vi "GetIndexInRange.vi"(8 "location":u32, 9 "buffer size":u32, 10 "last block":u32, 11 "write pointer":i32) -> (1 "index":i32, 2 "in range":bool)   [LabVIEW 2017, in "DVRBuffer.lvlib"]
uses:
  <vilib>/addons/InsightCM/Devices/Shared/Common/DVRBuffer/DVRBuffer.lvlib
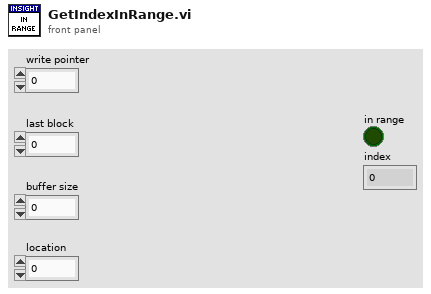
[diagram p1: front panel]
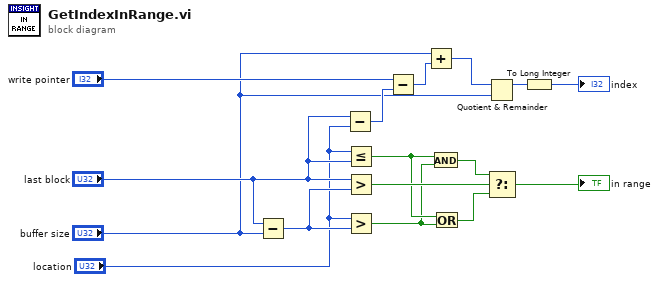
[diagram p0: block diagram]
diagram:
  n1 = Subtract(x="last block", y="buffer size") -> (x-y=w16:u32)
  n2 = Subtract(x="last block", y="location") -> (x-y=w14:u32)
  n3 = Less Or Equal?(x="location", y="last block") -> (x <= y?=w11:bool)
  n4 = Greater?(x="last block", y=w16) -> (0:w12:bool)
  n5 = Greater?(x="location", y=w16) -> (0:w10:bool)
  n6 = Subtract(x="write pointer", y=w14) -> (x-y=w3:u32)
  n7 = Add(x="buffer size", y=w3) -> (x+y=w1:u32)
  n8 = And(x=w11, y=w10) -> (x .and. y?=w8:bool)
  n9 = Or(x=w11, y=w10) -> (x .or. y?=w9:bool)
  n10 = Quotient & Remainder(x=w1, y="buffer size") -> (x-y*floor(x/y)=w13:u32)  [unwired: 1 out]
  n11 = Select(t=w8, s=w12, f=w9) -> (s? t:f=→"in range":bool)
  n12 = To Long Integer(number=w13) -> (32bit integer=→"index":i32)
